vi "VI Scripting Create Path From Template.vi"(4 "Reverse Path?":bool, 5 "Graph":cluster{dbl[], dbl[]}[](array[cluster]), 6 "VI in":refnum<vi>, 7 "Name":string, 9 "path":cluster{"X":dbl, "Y":dbl}[](array[cluster]), 10 "Data Points":T1[](array[typedef]), 11 "base path":path) -> ()   [LabVIEW 2018]
uses:
  Typedef/Data Point.ctl
  <vilib>/LabVIEW Icon API/API_Rectangle Dimension.ctl
  <vilib>/LabVIEW Icon API/API_Text.ctl
  <vilib>/LabVIEW Icon API/LabVIEW Icon API.lvlib
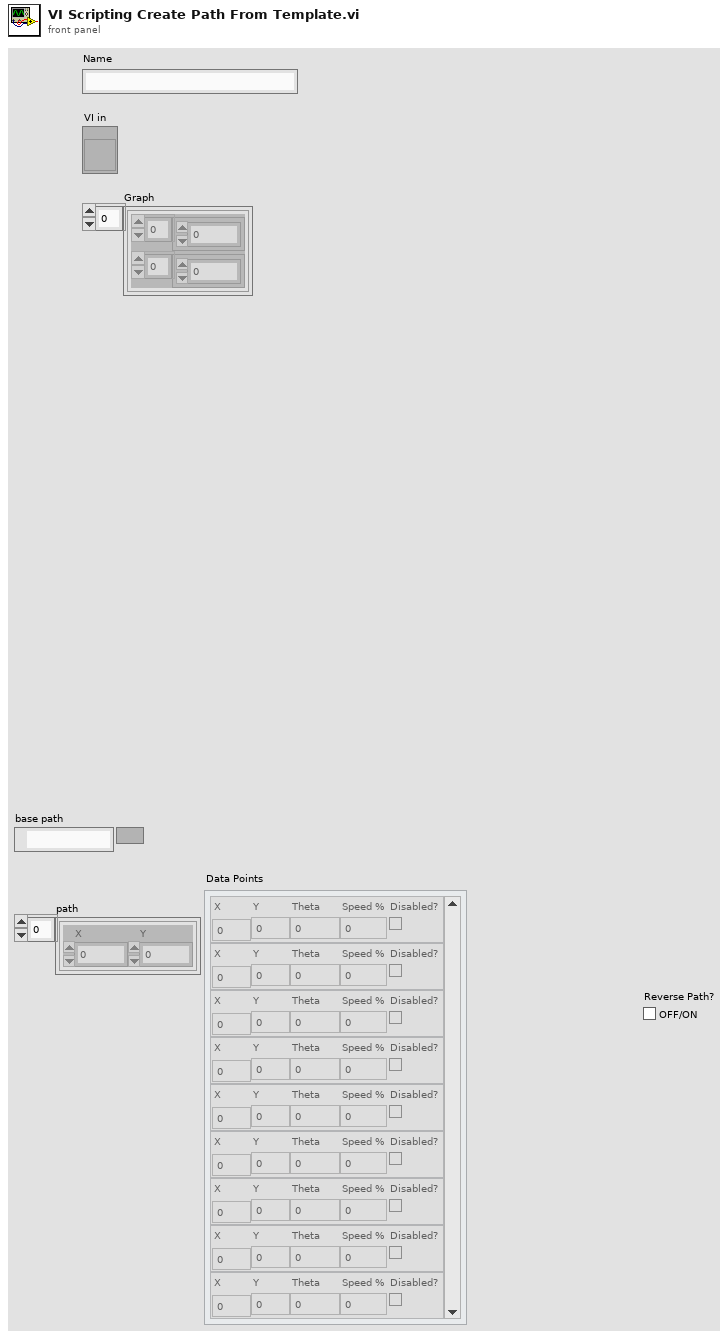
[diagram p1: front panel]
types:
  T1 = typedef "Data Point.ctl" = cluster{"X":dbl, "Y":dbl, "Theta":dbl, "Speed %":dbl, "Disabled?":bool}
  T2 = typedef "LabVIEW Icon API.lvlib/API_Text.ctl" = cluster{"Line 1 text":string, "Line 2 text":string, "Line 3 text":string, "Line 4 text":string}
  T3 = typedef "LabVIEW Icon API.lvlib/API_Rectangle Dimension.ctl" = cluster{"Width":i16, "Height":i16}
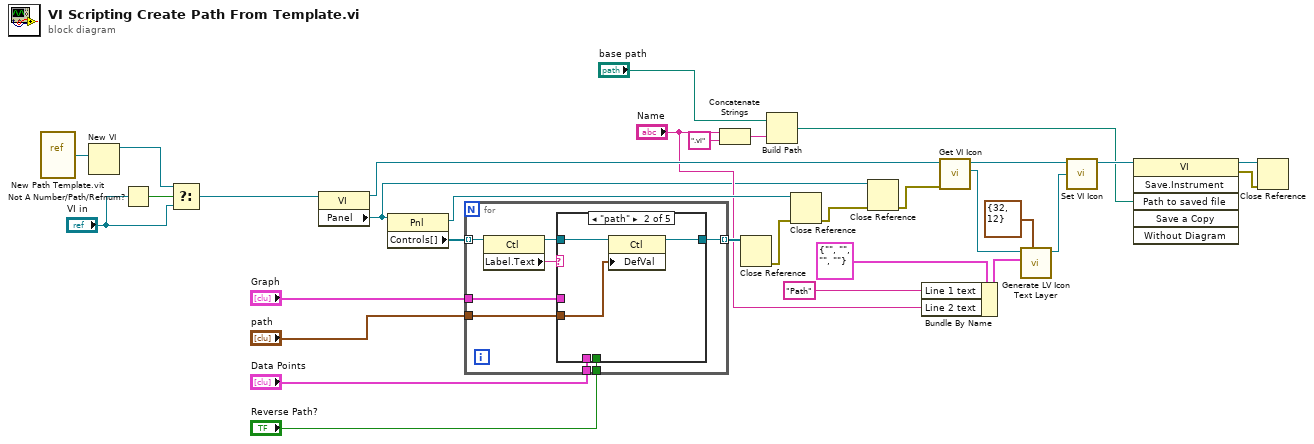
[diagram p0: block diagram]
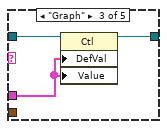
[diagram p3: hidden frame]
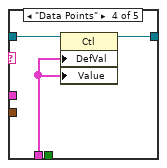
[diagram p4: hidden frame]
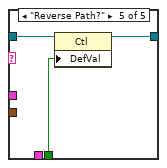
[diagram p5: hidden frame]
diagram:
  n1 = vi-ref "New Path Template.vit"() -> (w10:refnum<vi>)
  n2 = New VI(10:w10) -> (3:w12:refnum<vi>)  [unwired: 6 in, 1 out]
  n3 = Not A Number/Path/Refnum?(number/path/refnum="VI in") -> (NaN/Path/Refnum?=w9:bool)
  n4 = Select(t=w12, s=w9, f="VI in") -> (s? t:f=w11:refnum<vi>)
  n5 = property class="VI"(reference=w11) -> (reference out=w32:refnum<vi>, "Panel"=w15:refnum<vi>)  [unwired: 1 in, 1 out]
  n6 = property class="Pnl"(reference=w15) -> (reference out=w22:refnum<vi>, "Controls[]"=w18:refnum<vi>[])  [unwired: 1 in, 1 out]
  n7 = for {
    tunnel: w18 -> [w40] mode=indexing
    tunnel: "Graph" -> [w37]
    tunnel: [w36] -> w20 mode=indexing
    tunnel: "path" -> [w35]
    tunnel: "Data Points" -> [w34]
    tunnel: "Reverse Path?" -> [w33]
    n8 = property class="Ctl"(reference=w40) -> (reference out=w38:refnum<vi>, "Label.Text"=w39:string)  [unwired: 1 in, 1 out]
    n9 = case shown="\"path\"" w39 {
      tunnel: w38 -> [w41 w44 w47 w50 w53]
      tunnel: w37 -> [_ _ w45 _ _]
      tunnel: [w41 w43 w46 w49 w52] -> w36
      tunnel: w35 -> [_ w42 _ _ _]
      tunnel: w34 -> [_ _ _ w48 _]
      tunnel: w33 -> [_ _ _ _ w51]
      frame Default {
      }
      frame "path" {
        n10 = property class="Ctl"(reference=w44, "DefVal"=w42) -> (reference out=w43:refnum<vi>)  [unwired: 1 in, 1 out]
      }
      frame "Graph" {
        n11 = property class="Ctl"(reference=w47, "DefVal"=w45, "Value"=w45) -> (reference out=w46:refnum<vi>)  [unwired: 1 in, 1 out]
      }
      frame "Data Points" {
        n12 = property class="Ctl"(reference=w50, "DefVal"=w48, "Value"=w48) -> (reference out=w49:refnum<vi>)  [unwired: 1 in, 1 out]
      }
      frame "Reverse Path?" {
        n13 = property class="Ctl"(reference=w53, "DefVal"=w51) -> (reference out=w52:refnum<vi>)  [unwired: 1 in, 1 out]
      }
    }
  }
  n14 = Concatenate Strings("Name", ".vi" ("string")) -> (w23:string)
  n15 = Close Reference(reference=w20) -> (error out=w21:errorcluster)  [unwired: 1 in]
  n16 = Build Path(base path="base path", name or relative path=w23) -> (appended path=w6:path)
  n17 = Close Reference(reference=w22, error in (no error)=w21) -> (error out=w16:errorcluster)
  n18 = Close Reference(reference=w15, error in (no error)=w16) -> (error out=w14:errorcluster)
  n19 = Bundle By Name(cluster=T2 {"Line 1 text"="", "Line 2 text"="", "Line 3 text"="", "Line 4 text"=""} ("Text"), "Line 1 text"="Path", "Line 2 text"="Name") -> (w30:T2)
  n20 = call <vilib>:"Get VI Icon.vi"("error in (no error)"=w14, "VI Refnum in"=w32) -> ("Icon"=w26:refnum<class "Icon.lvclass">, "VI Refnum out"=w25:refnum<vi>)  [unwired: 7 in, 1 out]
  n21 = call <vilib>:"Generate LV Icon Text Layer.vi"("Rectangle dimension (32,32)"=T3 {"Width"=32, "Height"=12}, "Text"=w30, "Icon in"=w26) -> ("Icon out"=w27:refnum<class "Icon.lvclass">)  [unwired: 7 in, 1 out]
  n22 = call <vilib>:"Set VI Icon.vi"("Icon"=w27, "VI Refnum in"=w25) -> ("VI Refnum out"=w7:refnum<vi>)  [unwired: 8 in, 1 out]
  n23 = invoke class="VI" method="Save.Instrument"(reference=w7, "Path to saved file"=w6) -> (reference out=w8:refnum<vi>, error out=w3:errorcluster)  [unwired: 4 in, 4 out]
  n24 = Close Reference(reference=w8, error in (no error)=w3) -> ()  [unwired: 1 out]
